vi "ReadPhaseFromCalcCache.vi"(6 "calc cache":variant, 10 "channel name":string) -> (3 "phase":dbl, 4 "calc cache out":variant)   [LabVIEW 2017, in "AnalysisHelper.lvlib"]
uses:
  <vilib>/addons/InsightCM/Utilities/Analysis/Shared/AnalysisHelper.lvlib
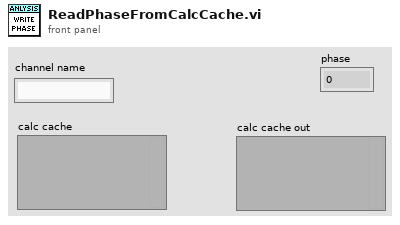
[diagram p1: front panel]
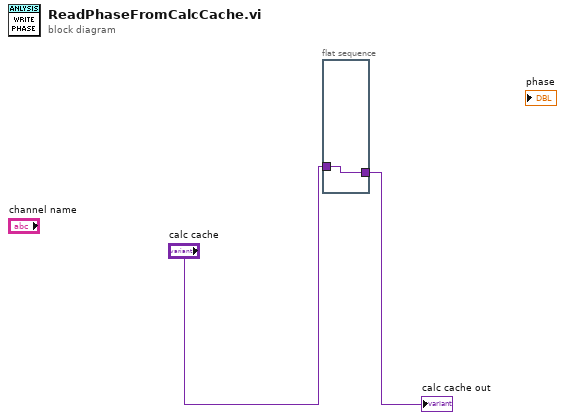
[diagram p0: block diagram]
diagram:
  n1 = flat-sequence {
    tunnel: [w3] -> w2
    tunnel: "calc cache" -> [w3]
    frame #0 {
    }
  }
  "calc cache out" <- w2
